vi "Mem1024.vi"(4 "Phi2":bool, 6 "Phi1":bool, 11 "Data In":bool) -> (3 "Data Out":bool)   [LabVIEW 2012]
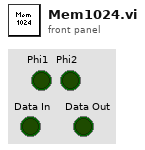
[diagram p1: front panel]
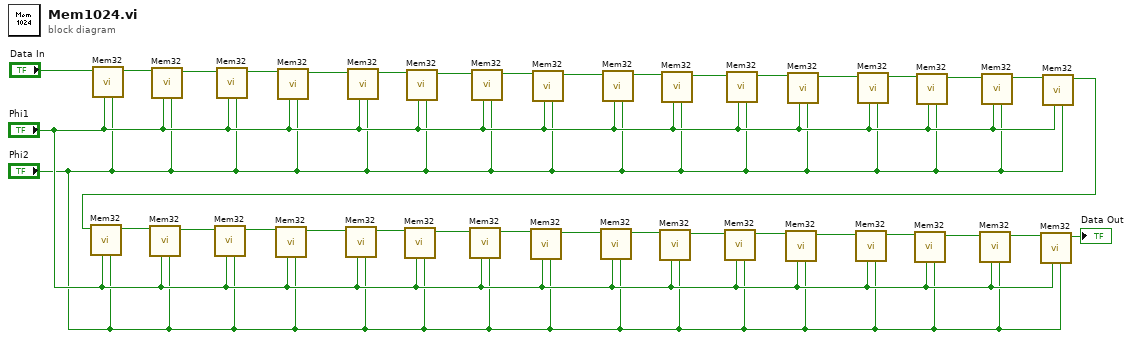
[diagram p0: block diagram]
diagram:
  n1 = call "Mem32.vi"("Phi1"="Phi2", "Phi0"="Phi1", "Data In"="Data In") -> ("Data Out"=w34:bool)  [unwired: 8 in]
  n2 = call "Mem32.vi"("Phi1"="Phi2", "Phi0"="Phi1", "Data In"=w34) -> ("Data Out"=w33:bool)  [unwired: 8 in]
  n3 = call "Mem32.vi"("Phi1"="Phi2", "Phi0"="Phi1", "Data In"=w33) -> ("Data Out"=w32:bool)  [unwired: 8 in]
  n4 = call "Mem32.vi"("Phi1"="Phi2", "Phi0"="Phi1", "Data In"=w32) -> ("Data Out"=w28:bool)  [unwired: 8 in]
  n5 = call "Mem32.vi"("Phi1"="Phi2", "Phi0"="Phi1", "Data In"=w28) -> ("Data Out"=w29:bool)  [unwired: 8 in]
  n6 = call "Mem32.vi"("Phi1"="Phi2", "Phi0"="Phi1", "Data In"=w29) -> ("Data Out"=w30:bool)  [unwired: 8 in]
  n7 = call "Mem32.vi"("Phi1"="Phi2", "Phi0"="Phi1", "Data In"=w30) -> ("Data Out"=w31:bool)  [unwired: 8 in]
  n8 = call "Mem32.vi"("Phi1"="Phi2", "Phi0"="Phi1", "Data In"=w31) -> ("Data Out"=w20:bool)  [unwired: 8 in]
  n9 = call "Mem32.vi"("Phi1"="Phi2", "Phi0"="Phi1", "Data In"=w20) -> ("Data Out"=w21:bool)  [unwired: 8 in]
  n10 = call "Mem32.vi"("Phi1"="Phi2", "Phi0"="Phi1", "Data In"=w21) -> ("Data Out"=w22:bool)  [unwired: 8 in]
  n11 = call "Mem32.vi"("Phi1"="Phi2", "Phi0"="Phi1", "Data In"=w22) -> ("Data Out"=w23:bool)  [unwired: 8 in]
  n12 = call "Mem32.vi"("Phi1"="Phi2", "Phi0"="Phi1", "Data In"=w23) -> ("Data Out"=w27:bool)  [unwired: 8 in]
  n13 = call "Mem32.vi"("Phi1"="Phi2", "Phi0"="Phi1", "Data In"=w27) -> ("Data Out"=w26:bool)  [unwired: 8 in]
  n14 = call "Mem32.vi"("Phi1"="Phi2", "Phi0"="Phi1", "Data In"=w26) -> ("Data Out"=w25:bool)  [unwired: 8 in]
  n15 = call "Mem32.vi"("Phi1"="Phi2", "Phi0"="Phi1", "Data In"=w25) -> ("Data Out"=w24:bool)  [unwired: 8 in]
  n16 = call "Mem32.vi"("Phi1"="Phi2", "Phi0"="Phi1", "Data In"=w24) -> ("Data Out"=w4:bool)  [unwired: 8 in]
  n17 = call "Mem32.vi"("Phi1"="Phi2", "Phi0"="Phi1", "Data In"=w4) -> ("Data Out"=w5:bool)  [unwired: 8 in]
  n18 = call "Mem32.vi"("Phi1"="Phi2", "Phi0"="Phi1", "Data In"=w5) -> ("Data Out"=w6:bool)  [unwired: 8 in]
  n19 = call "Mem32.vi"("Phi1"="Phi2", "Phi0"="Phi1", "Data In"=w6) -> ("Data Out"=w7:bool)  [unwired: 8 in]
  n20 = call "Mem32.vi"("Phi1"="Phi2", "Phi0"="Phi1", "Data In"=w7) -> ("Data Out"=w11:bool)  [unwired: 8 in]
  n21 = call "Mem32.vi"("Phi1"="Phi2", "Phi0"="Phi1", "Data In"=w11) -> ("Data Out"=w10:bool)  [unwired: 8 in]
  n22 = call "Mem32.vi"("Phi1"="Phi2", "Phi0"="Phi1", "Data In"=w10) -> ("Data Out"=w9:bool)  [unwired: 8 in]
  n23 = call "Mem32.vi"("Phi1"="Phi2", "Phi0"="Phi1", "Data In"=w9) -> ("Data Out"=w8:bool)  [unwired: 8 in]
  n24 = call "Mem32.vi"("Phi1"="Phi2", "Phi0"="Phi1", "Data In"=w8) -> ("Data Out"=w19:bool)  [unwired: 8 in]
  n25 = call "Mem32.vi"("Phi1"="Phi2", "Phi0"="Phi1", "Data In"=w19) -> ("Data Out"=w18:bool)  [unwired: 8 in]
  n26 = call "Mem32.vi"("Phi1"="Phi2", "Phi0"="Phi1", "Data In"=w18) -> ("Data Out"=w17:bool)  [unwired: 8 in]
  n27 = call "Mem32.vi"("Phi1"="Phi2", "Phi0"="Phi1", "Data In"=w17) -> ("Data Out"=w16:bool)  [unwired: 8 in]
  n28 = call "Mem32.vi"("Phi1"="Phi2", "Phi0"="Phi1", "Data In"=w16) -> ("Data Out"=w12:bool)  [unwired: 8 in]
  n29 = call "Mem32.vi"("Phi1"="Phi2", "Phi0"="Phi1", "Data In"=w12) -> ("Data Out"=w13:bool)  [unwired: 8 in]
  n30 = call "Mem32.vi"("Phi1"="Phi2", "Phi0"="Phi1", "Data In"=w13) -> ("Data Out"=w14:bool)  [unwired: 8 in]
  n31 = call "Mem32.vi"("Phi1"="Phi2", "Phi0"="Phi1", "Data In"=w14) -> ("Data Out"=w15:bool)  [unwired: 8 in]
  n32 = call "Mem32.vi"("Phi1"="Phi2", "Phi0"="Phi1", "Data In"=w15) -> ("Data Out"=→"Data Out":bool)  [unwired: 8 in]
